vi "ziOpen.vi"(3 "Error In":errorcluster, 4 "Port obsolete (auto)":u16, 5 "Hostname obsolete (auto)":string, 6 "Address":string="DEV") -> (0 "Error Out":errorcluster, 1 "Selected Device":string, 2 "HandleOut":T1 {"Handle" format="0x%08x"; "Conn" format="0x%08x"})   [LabVIEW 2016, in "Zurich Instruments LabOne.lvlib"]
doc: "Creates a connection to a Data Server. <b>Address</b> is of the format {<host>}{:<port}{::<Device ID>}. Usually it is sufficient to provide the <b>Device ID</b> only. The host and port are then determined by network discovery. Should the discovery not work, prepend <host>:<port>:: to the Device ID. Examples are \"myhf2.company.com:8004::dev466\" or \"myhf2.company.com:8004\". In the latter case the first found instrument on the data server listening on myhf2.company.com:8004 will be selected."
uses:
  Zurich Instruments LabOne.lvlib
  ziTypeHandle.ctl
  ziTypeDisovery.ctl
  <vilib>/Utility/error.llb/DialogType.ctl
  Private/ziLV64.dll
panel:
  out "auto-connected":bool
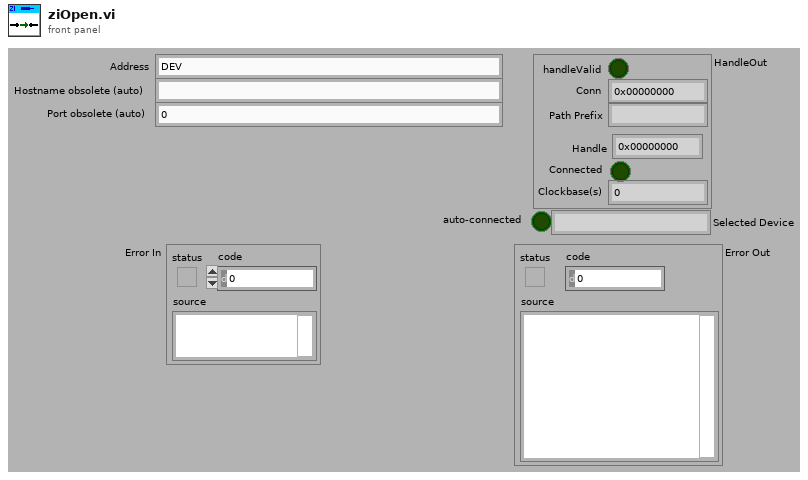
[diagram p1: front panel]
types:
  T1 = typedef "Zurich Instruments LabOne.lvlib/ziTypeHandle.ctl" = cluster{"handleValid":bool, "Conn":u64, "Path Prefix":string, "Handle":u64, "Connected":bool, "Clockbase(s)":dbl}
  T2 = typedef "ziTypeDisovery.ctl" = cluster{"timestamp":u64, "deviceid":string, "devicetype":string, "serveraddress":string, "serverport":u32, "apilevel":u32, "discoverable":bool, "interface":string, "connected":string, "available":bool, "owner":string, "status":string, "options ":string}
  T3 = typedef "DialogType.ctl" = u16
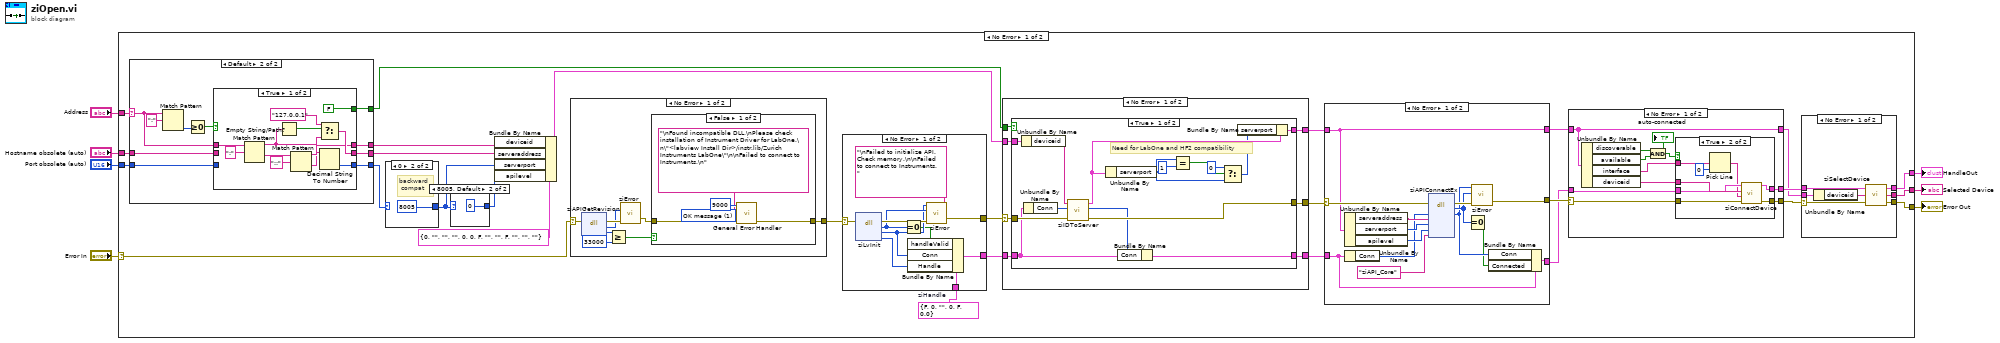
[diagram p0: block diagram]
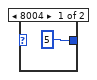
[diagram p2: hidden frame]
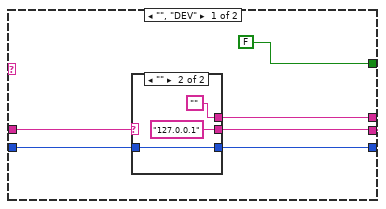
[diagram p4: hidden frame]
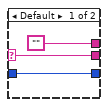
[diagram p5: hidden frame]
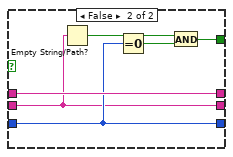
[diagram p6: hidden frame]
diagram:
  n1 = case shown="No Error" "Error In" {
    selector: "Error In" -> [w26 w185]
    tunnel: [w35 w185] -> w7
    tunnel: [w34 _] -> w6
    tunnel: "Hostname obsolete (auto)" -> [w24 _]
    tunnel: "Port obsolete (auto)" -> [w25 _]
    tunnel: [w33 _] -> w3
    tunnel: "Address" -> [w23 _]
    frame No Error {
      w12 = T1 {"handleValid"=FALSE, "Conn"=0, "Path Prefix"="", "Handle"=0, "Connected"=FALSE, "Clockbase(s)"=0.0}  # ziHandle
      n2 = case shown="Default" w23 {
        selector: w23 -> [_ w54]
        tunnel: w24 -> [w45 w60]
        tunnel: w25 -> [w44 w56]
        tunnel: [w43 w61] -> w17
        tunnel: [w42 w59] -> w14
        tunnel: [w41 w58] -> w13
        tunnel: [FALSE w57] -> w8
        frame "", "DEV" {
          n3 = case shown="\"\"" w45 {
            selector: w45 -> [w47 _]
            tunnel: w44 -> [w46 w51]
            tunnel: [w46 w51] -> w43
            tunnel: [w47 "127.0.0.1"] -> w42
            tunnel: ["" ""] -> w41
            frame Default {
            }
            frame "" {
            }
          }
        }
        frame Default {
          n4 = Match Pattern(string=w54, regular expression=":") -> (offset past match=w55:i32)  [unwired: 1 in, 3 out]
          n5 = Greater Or Equal To 0?(x=w55) -> (x >= 0?=w52:bool)
          n6 = case shown="True" w52 {
            tunnel: [w66 w78] -> w61
            tunnel: w60 -> [_ w75]
            tunnel: [w68 w75] -> w59
            tunnel: w54 -> [w72 w79]
            tunnel: [w65 w79] -> w58
            tunnel: [FALSE w76] -> w57
            tunnel: w56 -> [_ w78]
            frame True {
              n7 = Match Pattern(string=w72, regular expression=":") -> (before substring=w63:string, after substring=w69:string)  [unwired: 1 in, 2 out]
              n8 = Empty String/Path?(string/path=w63) -> (empty?=w62:bool)
              n9 = Match Pattern(string=w69, regular expression="::") -> (before substring=w67:string, after substring=w65:string)  [unwired: 1 in, 2 out]
              n10 = Select(t="127.0.0.1", s=w62, f=w63) -> (s? t:f=w68:string)
              n11 = Decimal String To Number(string=w67) -> (number=w66:i32)  [unwired: 2 in, 1 out]
            }
            frame False {
              n12 = Empty String/Path?(string/path=w75) -> (empty?=w74:bool)
              n13 = Equal To 0?(x=w78) -> (x = 0?=w77:bool)
              n14 = And(x=w74, y=w77) -> (x .and. y?=w76:bool)
            }
          }
        }
      }
      n15 = case shown="0" w17 {
        selector: w17 -> [w38 _]
        tunnel: [w38 8005] -> w15
        frame Default {
        }
        frame 0 {
          # "backward\n compat"
        }
      }
      n16 = case shown="8005, Default" w15 {
        tunnel: [5 0] -> w16
        frame 8004 {
        }
        frame 8005, Default {
        }
      }
      n17 = Bundle By Name(cluster=T2 {"timestamp"=0, "deviceid"="", "devicetype"="", "serveraddress"="", "serverport"=0, "apilevel"=0, "discoverable"=FALSE, "interface"="", "connected"="", "available"=FALSE, "owner"="", "status"="", "options "=""} ("ziDiscovery"), "deviceid"=w13, "serveraddress"=w14, "serverport"=w15, "apilevel"=w16) -> (w19:T2)
      n18 = case shown="No Error" w26 {
        selector: w26 -> [w154 w167]
        tunnel: [w157 w167] -> w29
        frame No Error {
          n19 = dll-call lib="C:/Users/putkonen.CPFS/Desktop/resonant_ultrasound_arxiv/maglab ultrasound -- arkady --arxiv/Zurich/Zurich Instruments/LabOne/API/LabVIEW/Zurich Instruments LabOne/Private/ziLV*.*" fn="ziAPIGetRevision" label="GetRev"(error in=w154) -> (error out=w156:errorcluster, "return type"=w155:u32, "rev"=w160:u32)  [unwired: 2 in, 2 out]
          n20 = Greater Or Equal?(x=w160, y=u32 33000 ("rev")) -> (x >= y?=w158:bool)
          n21 = call "ziError.vi"("ziErrorCode"=w155, "Error In"=w156) -> ("Error Out"=w153:errorcluster)  [unwired: 4 in]
          n22 = case shown="False" w158 {
            tunnel: [w163 w166] -> w157
            tunnel: w153 -> [w165 w166]
            frame False {
              w164 = T3 1 items=["no dialog", "OK message", "continue or stop message", "OK message + warnings", "continue/stop + warnings"] ("type of dialog (OK msg:1)")
              n23 = call <vilib>:"General Error Handler.vi"("[error code] (0)"=9000, "[error source] (\" \")"="\nFound incompatible DLL.\nPlease check installation of Instrument Driver for LabOne.\n\"<labview Install Dir>/instr.lib/Zurich Instruments LabOne\"\n\nFailed to connect to Instruments.\n" ("message"), "type of dialog (OK msg:1)"=w164, "error in (no error)"=w165) -> ("error out"=w163:errorcluster)  [unwired: 7 in, 4 out]
            }
            frame True {
            }
          }
        }
        frame Error {
        }
      }
      n24 = case shown="No Error" w29 {
        selector: w29 -> [w118 w124]
        tunnel: [w119 w124] -> w28
        tunnel: w12 -> [w114 w123]
        tunnel: [w113 w123] -> w11
        frame No Error {
          n25 = dll-call lib="C:/Users/putkonen.CPFS/Desktop/resonant_ultrasound_arxiv/maglab ultrasound -- arkady --arxiv/Zurich/Zurich Instruments/LabOne/API/LabVIEW/Zurich Instruments LabOne/Private/ziLV*.*" fn="ziLvInit"(error in=w118) -> (error out=w122:errorcluster, "return type"=w120:u32, "Conn"=w116:u64, "ziLVHandle"=w117:u64)  [unwired: 2 in, 3 out]
          n26 = Equal To 0?(x=w120) -> (x = 0?=w115:bool)
          n27 = Bundle By Name(cluster=w114, "handleValid"=w115, "Conn"=w116, "Handle"=w117) -> (w113:T1)
          n28 = call "ziError.vi"("Conn"=w116, "ziErrorCode"=w120, "Error In"=w122, "Annotation"="\nFailed to initialize API. Check memory.\n\nFailed to connect to Instruments." ("message")) -> ("Error Out"=w119:errorcluster)  [unwired: 2 in]
        }
        frame Error {
        }
      }
      n29 = case shown="No Error" w28 {
        selector: w28 -> [w131 w152]
        tunnel: [w130 w152] -> w27
        tunnel: [w129 w150] -> w22
        tunnel: w8 -> [w128 _]
        tunnel: w19 -> [w127 w150]
        tunnel: w11 -> [w126 w151]
        tunnel: [w125 w151] -> w10
        frame No Error {
          n30 = case shown="True" w128 {
            tunnel: w131 -> [w146 w149]
            tunnel: [w145 w149] -> w130
            tunnel: [w143 w148] -> w129
            tunnel: w127 -> [w137 w148]
            tunnel: w126 -> [w133 w147]
            tunnel: [w134 w147] -> w125
            frame True {
              # "Need for LabOne and HF2 compatibility"
              n31 = Unbundle By Name(w137) -> ("deviceid"=w136:string)
              n32 = Unbundle By Name(w133) -> ("Conn"=w132:u64)
              n33 = call "ziIDToServer.vi"("Error In"=w146, "Conn In"=w132, "Device ID"=w136) -> ("Error Out"=w145:errorcluster, "Conn Out"=w135:u64, "ziDiscovery"=w144:T2)  [unwired: 6 in]
              n34 = Unbundle By Name(w144) -> ("serverport"=w139:u32)
              n35 = Bundle By Name(cluster=w133, "Conn"=w135) -> (w134:T1)
              n36 = Equal?(x=w139, y=u32 1) -> (x = y?=w141:bool)
              n37 = Select(t=u64 0, s=w141, f=w139) -> (s? t:f=w138:u64)
              n38 = Bundle By Name(cluster=w144, "serverport"=w138) -> (w143:T2)
            }
            frame False {
            }
          }
        }
        frame Error {
        }
      }
      n39 = case shown="No Error" w27 {
        selector: w27 -> [w177 w184]
        tunnel: [w180 w184] -> w30
        tunnel: w22 -> [w174 w183]
        tunnel: [w174 w183] -> w21
        tunnel: w10 -> [w170 w182]
        tunnel: [w168 w182] -> w9
        frame No Error {
          n40 = Unbundle By Name(w174) -> ("serveraddress"=w176:string, "serverport"=w175:u32, "apilevel"=w173:u32)
          n41 = Unbundle By Name(w170) -> ("Conn"=w172:u64)
          n42 = dll-call lib="C:/Users/putkonen.CPFS/Desktop/resonant_ultrasound_arxiv/maglab ultrasound -- arkady --arxiv/Zurich/Zurich Instruments/LabOne/API/LabVIEW/Zurich Instruments LabOne/Private/ziLV*.*" fn="ziAPIConnectEx"(error in=w177, "Conn"=w172, "hostname"=w176, "Port"=w175, "ZIAPIVersion_enum"=w173, "Implementation"="ziAPI_Core") -> (error out=w181:errorcluster, "return type"=w179:u32, "Conn"=w171:u64)  [unwired: 6 in, 1 out]
          n43 = Equal To 0?(x=w179) -> (x = 0?=w169:bool)
          n44 = call "ziError.vi"("Conn"=w171, "ziErrorCode"=w179, "Error In"=w181) -> ("Error Out"=w180:errorcluster)  [unwired: 3 in]
          n45 = Bundle By Name(cluster=w170, "Conn"=w171, "Connected"=w169) -> (w168:T1)
        }
        frame Error {
        }
      }
      n46 = case shown="No Error" w30 {
        selector: w30 -> [w94 w111]
        tunnel: w21 -> [w90 w110]
        tunnel: w9 -> [w98 w112]
        tunnel: [w97 w112] -> w32
        tunnel: [w96 w111] -> w31
        tunnel: [w90 w110] -> w20
        frame No Error {
          n47 = Unbundle By Name(w90) -> ("discoverable"=w92:bool, "available"=w93:bool, "interface"=w95:string, "deviceid"=w99:string)
          n48 = And(x=w92, y=w93) -> (x .and. y?=w91:bool)
          "auto-connected" <- w91
          n49 = case shown="True" w91 {
            tunnel: w99 -> [_ w109]
            tunnel: w98 -> [w100 w105]
            tunnel: [w100 w108] -> w97
            tunnel: [w101 w107] -> w96
            tunnel: w95 -> [_ w103]
            tunnel: w94 -> [w101 w106]
            frame False {
            }
            frame True {
              n50 = Pick Line(multi-line string=w103, line index=0) -> (output string=w104:string)  [unwired: 1 in]
              n51 = call "ziConnectDevice.vi"("Error In"=w106, "Device Interface"=w104, "Device Serial"=w109, "Handle In"=w105) -> ("Error Out"=w107:errorcluster, "Handle Out"=w108:T1)  [unwired: 6 in]
            }
          }
        }
        frame Error {
        }
      }
      n52 = case shown="No Error" w31 {
        selector: w31 -> [w82 w87]
        tunnel: [w86 w87] -> w35
        tunnel: w32 -> [w83 w89]
        tunnel: [w84 w89] -> w34
        tunnel: [w85 ""] -> w33
        tunnel: w20 -> [w81 _]
        frame No Error {
          n53 = Unbundle By Name(w81) -> ("deviceid"=w80:string)
          n54 = call "ziSelectDevice.vi"("Error In"=w82, "Device (first)"=w80, "Handle In"=w83) -> ("Error Out"=w86:errorcluster, "Selected Device"=w85:string, "Handle Out"=w84:T1)
        }
        frame Error {
        }
      }
    }
    frame Error {
    }
  }
  "Error Out" <- w7
  "HandleOut" <- w6
  "Selected Device" <- w3
